vi "NBFM Modulation Demo (Single Tone) -  Template.vi"() -> ()   [LabVIEW 2013]
panel:
  in  "Mod. Freq.":dbl=2000.0 caption="Frequency"
  in  "WAV SR":dbl=44100.0 caption="dt"
  in  "LPF Cut-Off":dbl=5000.0 caption="Lower Cut-Off"
  in  "AWGN (dB)":dbl(slide)=30.0 caption="Standard deviation" scale=-20.0..50.0
  out "Recovered Signal":dynamicdata(graph)
  out "Baseband":dynamicdata(graph)
  out "FM FFT":dynamicdata(graph)
  out "FM Wave":dynamicdata(graph)
  in  "Carrier Amp.":dbl=1.0 caption="Amplitude"
  in  "stop":bool
  in  "Frequency Deviation":dbl(slide)=200.0 scale=0.0..400.0
  in  "Carrier Freq.":dbl=100000.0 caption="Frequency"
  # "Frequency Modulation"
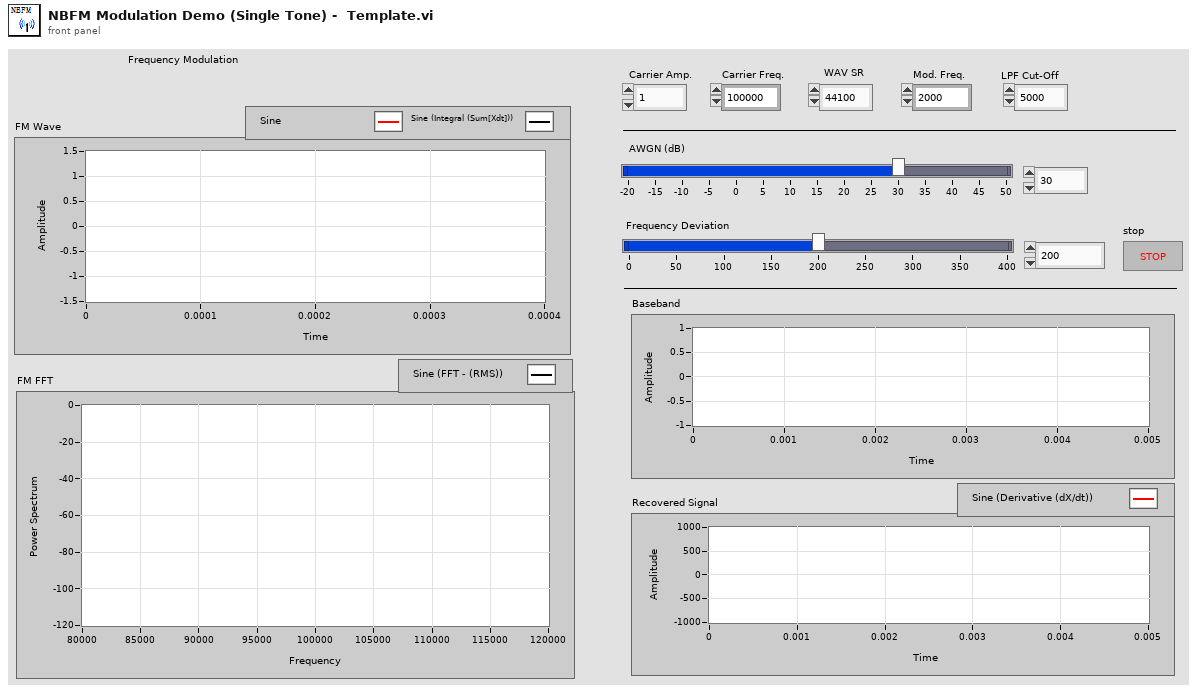
[diagram p1: front panel]
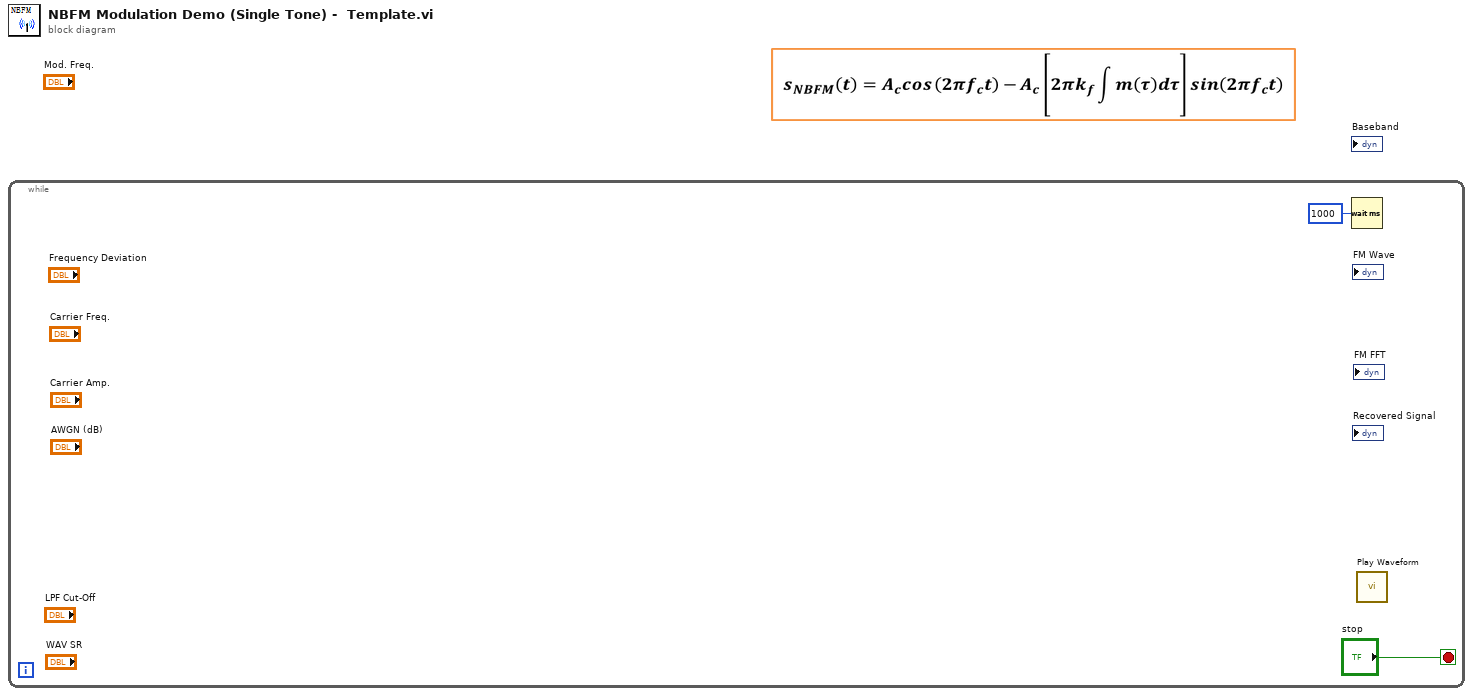
[diagram p0: block diagram]
diagram:
  n1 = while {
    stop <- "stop" stop-if-true
    n2 = Wait (ms)(milliseconds to wait=u32 1000) -> ()  [unwired: 1 out]
    n3 = call "Play Waveform"() -> ()  [unwired: 19 in, 1 out]
  }
